vi "instr_destroy.vi"(8 "error in (no error)":errorcluster, 11 "Instrument in":refnum<class "Instrument.lvclass">) -> (0 "error out":errorcluster)   [LabVIEW 2019, in "Instrument.lvclass"]
uses:
  Instrument.lvclass
  Instrument.lvclass/Instrument.ctl
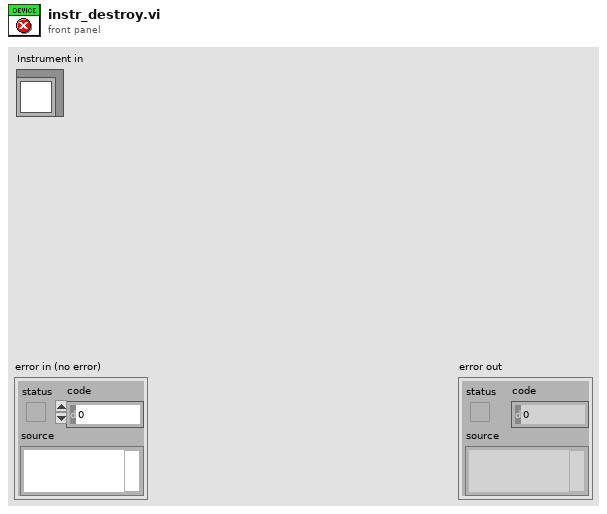
[diagram p1: front panel]
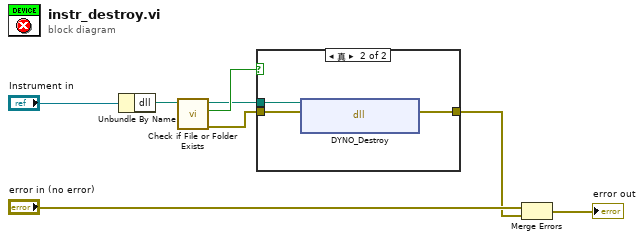
[diagram p0: block diagram]
diagram:
  n1 = Unbundle By Name("Instrument in") -> ("dll"=w6:path)
  n2 = call <vilib>:"Check if File or Folder Exists.vi"("path"=w6) -> ("error out"=w3:errorcluster, "file or folder exists?"=w5:bool, "dup path"=w4:path)  [unwired: 8 in]
  n3 = case shown="真" w5 {
    tunnel: w4 -> [_ w12]
    tunnel: w3 -> [w9 w11]
    tunnel: [w9 w10] -> w1
    frame False {
    }
    frame True {
      n4 = dll-call lib="C:/Dev/22KW-Dyno/software/data/DynoAPI.dll" fn="DYNO_Destroy"(path in=w12, error in=w11) -> (error out=w10:errorcluster)  [unwired: 2 in, 1 out]
    }
  }
  n5 = Merge Errors("error in (no error)", w1) -> (→"error out":errorcluster)
